vi "from string.vi"(8 "error in":errorcluster, 9 "data":string, 10 "version":string, 11 "Digitizer configuration":refnum<class "Digitizer configuration.lvclass">) -> (0 "error out":errorcluster, 3 "Digitizer configuration out":refnum<class "Digitizer configuration.lvclass">)   [LabVIEW 2025, in "Digitizer.lvlib" / "Digitizer configuration.lvclass"]
doc: "Provides an interface for loading a module configuration from a file or other serialized data source. It is recommended that all children of this class store data in two sets--data required for its own initialization, and any data required for parent initialization--and that each implementation uses the <b>Call Parent Method</b> primitive to de-serialize parent information.Copyright 2017 National Instruments Corporation\n\nLicensed under the Apache License, Version 2.0 (the \"License\"); you may not use this file except in compliance with the License. You may obtain a copy of the License at http://www.apache.org/licenses/LICENSE-2.0\nUnless required by applicable law or agreed to in writing, software distributed under the License is distributed on an \"AS IS\" BASIS, WITHOUT WARRANTIES OR CONDITIONS OF ANY KIND, either express or implied. See the License for the specific language governing permissions and limitations under the License."
uses:
  Digitizer configuration.lvclass
  Digitizer Instrument Setting.ctl
  Digitizer configuration.lvclass/Digitizer configuration.ctl
  Users/Public/Documents/Sandia National Labs/TSS Plugin/Abstract Engine.lvlibp/Instrument configuration/Instrument configuration.lvclass
  Users/Public/Documents/Sandia National Labs/TSS Plugin/CEF.lvlibp/serializable configuration/CEF_serializable configuration.lvclass
  Users/Public/Documents/Sandia National Labs/TSS Plugin/CEF.lvlibp
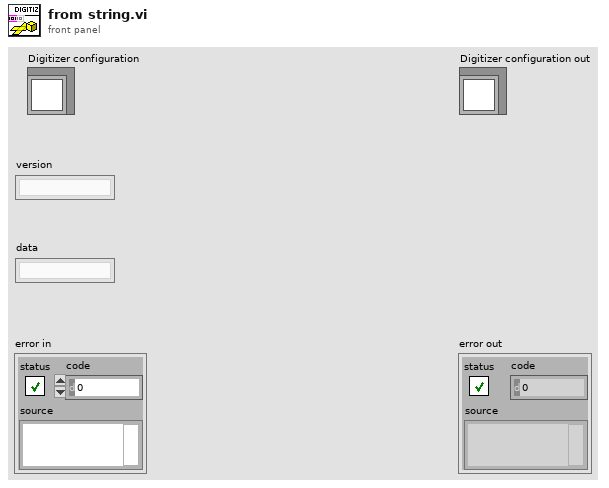
[diagram p1: front panel]
types:
  T1 = typedef "Digitizer.lvlib/Digitizer configuration.lvclass/Digitizer Instrument Setting.ctl" = cluster{"SampleMode":string, "SampleDuration":dbl, "SampleRate":u32, "ReferenceClock":string, "SampleClockEdge":string, "TrigType":string, "TrigLevel":dbl, "TrigSource":string, "Pretrigger":dbl, "TrigDest":string}
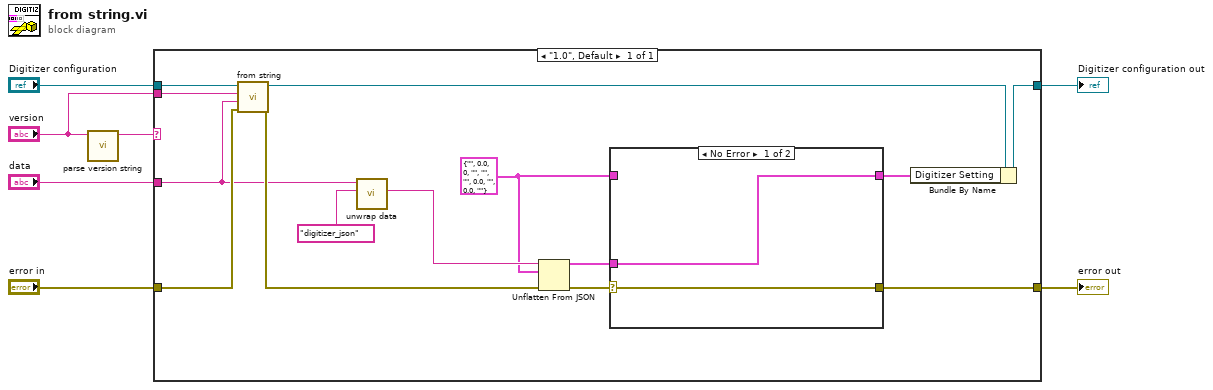
[diagram p0: block diagram]
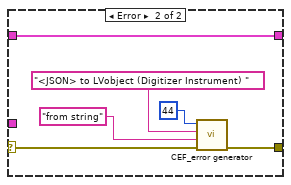
[diagram p2: hidden frame]
diagram:
  n1 = call "parse version string.vi"("full version"="version") -> ("major.minor version"=w3:string)  [unwired: 7 in, 3 out]
  n2 = case shown="\"1.0\", Default" w3 {
    tunnel: "Digitizer configuration" -> [w21]
    tunnel: [w16] -> w4
    tunnel: "data" -> [w13]
    tunnel: "error in" -> [w18]
    tunnel: "version" -> [w14]
    tunnel: [w11] -> w1
    frame "1.0", Default {
      w10 = T1 {"SampleMode"="", "SampleDuration"=0.0, "SampleRate"=0, "ReferenceClock"="", "SampleClockEdge"="", "TrigType"="", "TrigLevel"=0.0, "TrigSource"="", "Pretrigger"=0.0, "TrigDest"=""} ("Setting")
      n3 = call-parent "from string.vi"("error in"=w18, "data"=w13, "version"=w14, "Instrument configuration"=w21) -> ("error out"=w15:errorcluster, "Instrument configuration out"=w20:refnum<class "Digitizer configuration.lvclass">)  [unwired: 6 in]
      n4 = call "unwrap data.vi"("identifier"="digitizer_json" ("additional identifier"), "data to unwrap"=w13) -> ("unwrapped data"=w17:string)  [unwired: 8 in, 1 out]
      n5 = Unflatten From JSON(JSON string=w17, type and defaults=w10, error in (no error)=w15) -> (value=w9:T1, error out=w12:errorcluster)  [unwired: 4 in]
      n6 = case shown="No Error" w12 {
        selector: w12 -> [w22 w26]
        tunnel: w9 -> [w23 _]
        tunnel: [w23 w25] -> w8
        tunnel: w10 -> [_ w25]
        tunnel: [w22 w24] -> w11
        frame No Error {
        }
        frame Error {
          n7 = call "CEF_error generator.vi"("error in"=w26, "source"="from string" ("message"), "append error message"="<JSON> to LVobject (Digitizer Instrument) " ("message"), "error code (0)"=44) -> ("error out"=w24:errorcluster)  [unwired: 5 in]
        }
      }
      n8 = Bundle By Name(cluster=w20, "Digitizer Setting"=w8) -> (w16:refnum<class "Digitizer configuration.lvclass">)
    }
  }
  "error out" <- w1
  "Digitizer configuration out" <- w4
